vi "GetPatternMatchResultValue.vi"(8 "error in (no error)":errorcluster, 9 "PatternMatchResult":T1 {"results"."ROI Descriptor out"."Contours"."Type" items=["No Selection", "Point", "Line", "Rectangle", "Oval", "Polygon", "Freehand Region", "Annulus", "Unused2", "Unused3", "Broken Line", "Freehand Line", "Rotated Rectangle"]; "results"."Point"."Y" format="%.2f"; "results"."Point"."X" format="%.2f"; "results"."Rectangle"."Rotation" format="%.2f"; "results"."Rectangle"."Left" scale=0.0..1024.0; "results"."Rectangle"."Right" scale=0.0..1024.0}, 11 "PatternMatchParameter":T5={"Algorithm"=2, "Match Parameters"={"Number of Matches Requested"=1, "Minimum Match Score"=750.0, "Angle Ranges"=[]}, "ROI Descriptor"={"Global Rectangle"=[], "Contours"=[]}, "Advanced Options"=[{"Item"=1, "Value"=1.0}, {"Item"=103, "Value"=1.0}], "Template path"="", "XOffset"=0, "YOffset"=0} {"ROI Descriptor"."Contours"."Type" items=["No Selection", "Point", "Line", "Rectangle", "Oval", "Polygon", "Freehand Region", "Annulus", "Unused2", "Unused3", "Broken Line", "Freehand Line", "Rotated Rectangle"]; "Advanced Options"."Item" items=["LD Sampling - Minimum Constrast"=0, "LD Sampling - Enable Subpixel Accuracy"=1, "LD Sampling - Search Strategy"=2, "LD Sampling - Subpixel Iterations"=3, "LD Sampling - Subpixel Tolerance"=4, "LD Sampling - Initial Match List Length"=5, "LD Sampling - Match List Reduction Factor"=6, "LD Sampling - Initial Step Size"=7, "LD Sampling - Intermediate Angular Accuracy"=8, "-"=9, "Pyramid - Max Pyramid Level"=100, "Pyramid - Minimum Contrast"=102, "Pyramid - Enable Subpixel Accuracy"=103, "Pyramid - Subpixel Iterations"=104, "Pyramid - Subpixel Tolerance"=105, "Pyramid - Initial Match List Length"=106, "Pyramid - Match List Reduction Factor"=107, "Pyramid - Intermediate Angular Accuracy"=108, "Pyramid - Process Border Matches"=109, "Pyramid - Min Match Separation Distance"=111, "Pyramid - Min Match Separation Angle"=112, "Pyramid - Max Match Overlap"=113, "Pyramid - Max Cache in MB"=114, "Pyramid - Clear Cache"=115]; "Match Parameters"."Angle Ranges"."End Angle" min=-360 max=360; "Match Parameters"."Angle Ranges"."Start Angle" min=-360 max=360; "Match Parameters"."Minimum Match Score" min=0 max=1000; "Match Parameters"."Number of Matches Requested" min=1 max=9999; "Algorithm" items=["All", "Low Discrepancy Sampling", "Grayscale Value Pyramid", "Gradients Pyramid"]}) -> (0 "error out":errorcluster, 3 "ResultValues":string[](array[string]))   [LabVIEW 2019]
uses:
  Controls/Parttern Match/Analysis_PatternMatch_Parameter.ctl
  Controls/Parttern Match/Analysis_PatternMatch_ResultWithnumber.ctl
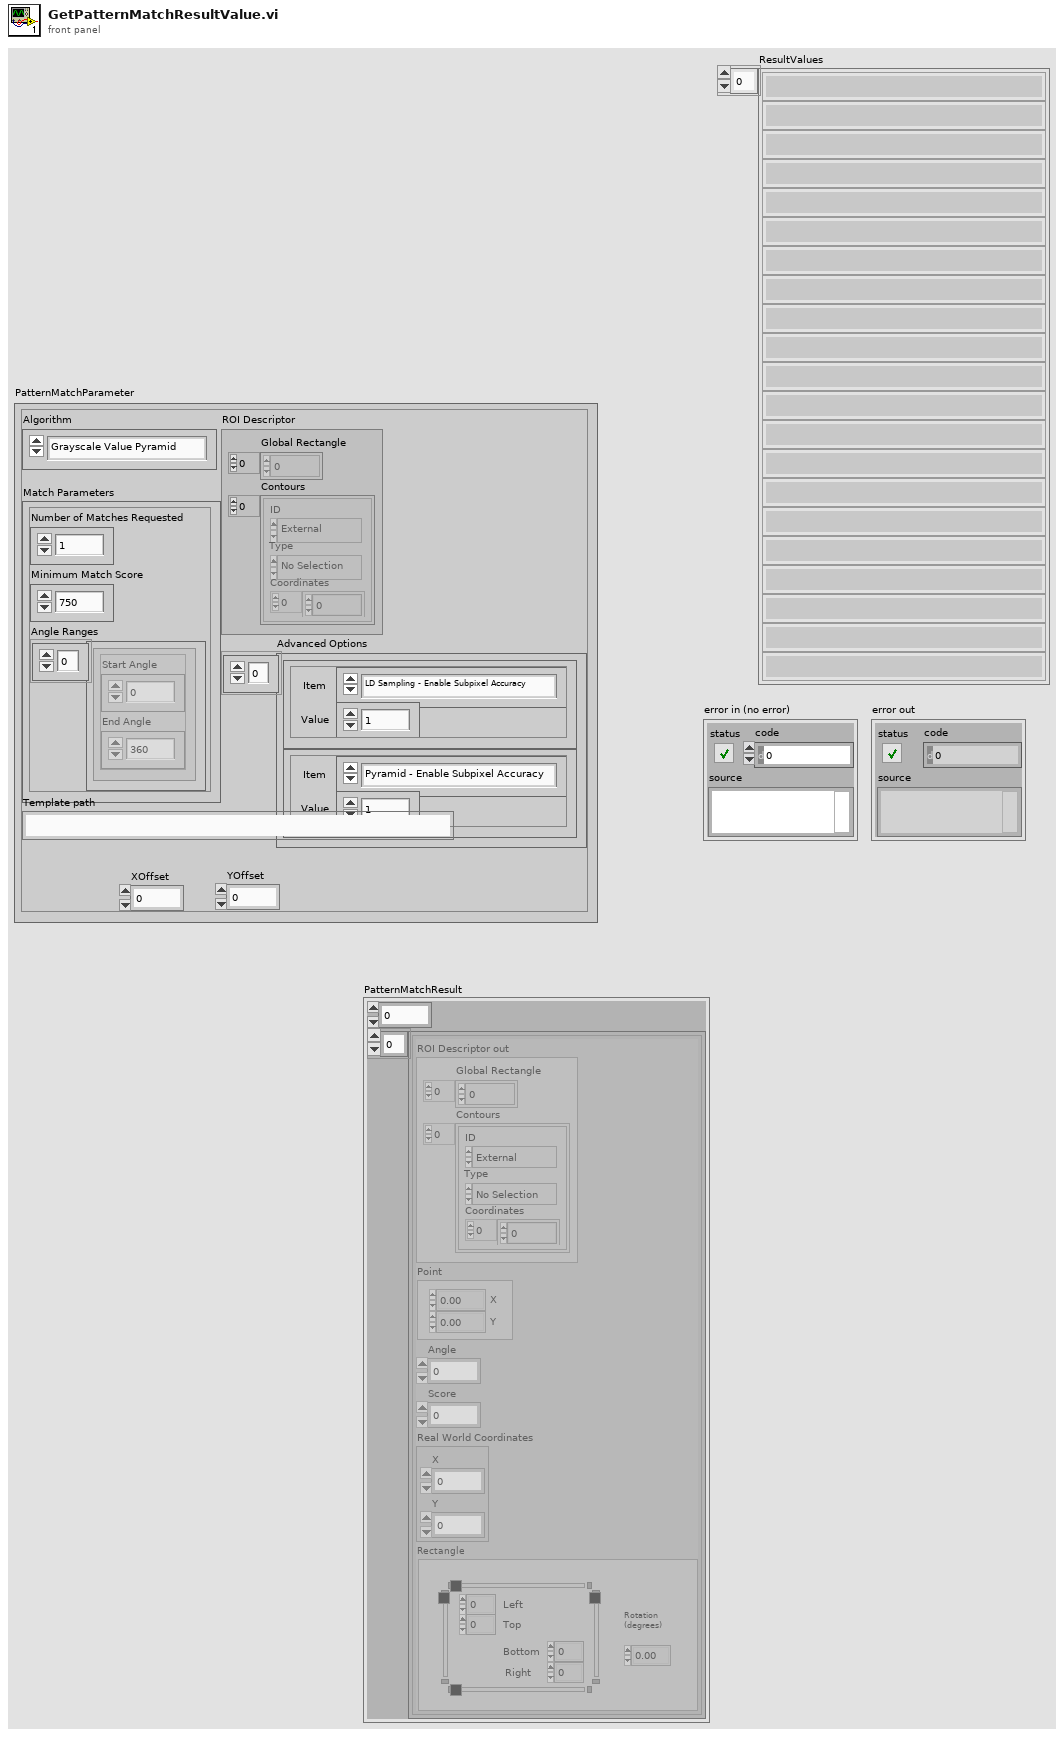
[diagram p1: front panel]
types:
  T1 = typedef "Analysis_PatternMatch_ResultWithnumber.ctl" = cluster{"numbers":i32, "results":cluster{"ROI Descriptor out":T2, "Point":T3, "Angle":sgl, "Score":sgl, "Real World Coordinates":cluster{"X":sgl, "Y":sgl}, "Rectangle":T4}[]}
  T2 = typedef "ROI Descriptor" = cluster{"Global Rectangle":i32[], "Contours":cluster{"ID":enum32{"External", "Internal"}, "Type":u32, "Coordinates":i32[]}[]}
  T3 = typedef "IMAQ Point" = cluster{"X":sgl, "Y":sgl}
  T4 = typedef "IMAQ Rectangle" = cluster{"Left":i32, "Top":i32, "Right":i32, "Bottom":i32, "Rotation":dbl}
  T5 = typedef "Analysis_PatternMatch_Parameter.ctl" = cluster{"Algorithm":i32, "Match Parameters":cluster{"Number of Matches Requested":i32, "Minimum Match Score":sgl, "Angle Ranges":cluster{"Start Angle":sgl, "End Angle":sgl}[]}, "ROI Descriptor":T2, "Advanced Options":cluster{"Item":u16, "Value":dbl}[], "Template path":string, "XOffset":i32, "YOffset":i32}
  T6 = cluster{"ROI Descriptor out":T2, "Point":T3, "Angle":sgl, "Score":sgl, "Real World Coordinates":cluster{"X":sgl, "Y":sgl}, "Rectangle":T4}[]
  T7 = cluster{"ROI Descriptor out":T2, "Point":T3, "Angle":sgl, "Score":sgl, "Real World Coordinates":cluster{"X":sgl, "Y":sgl}, "Rectangle":T4}
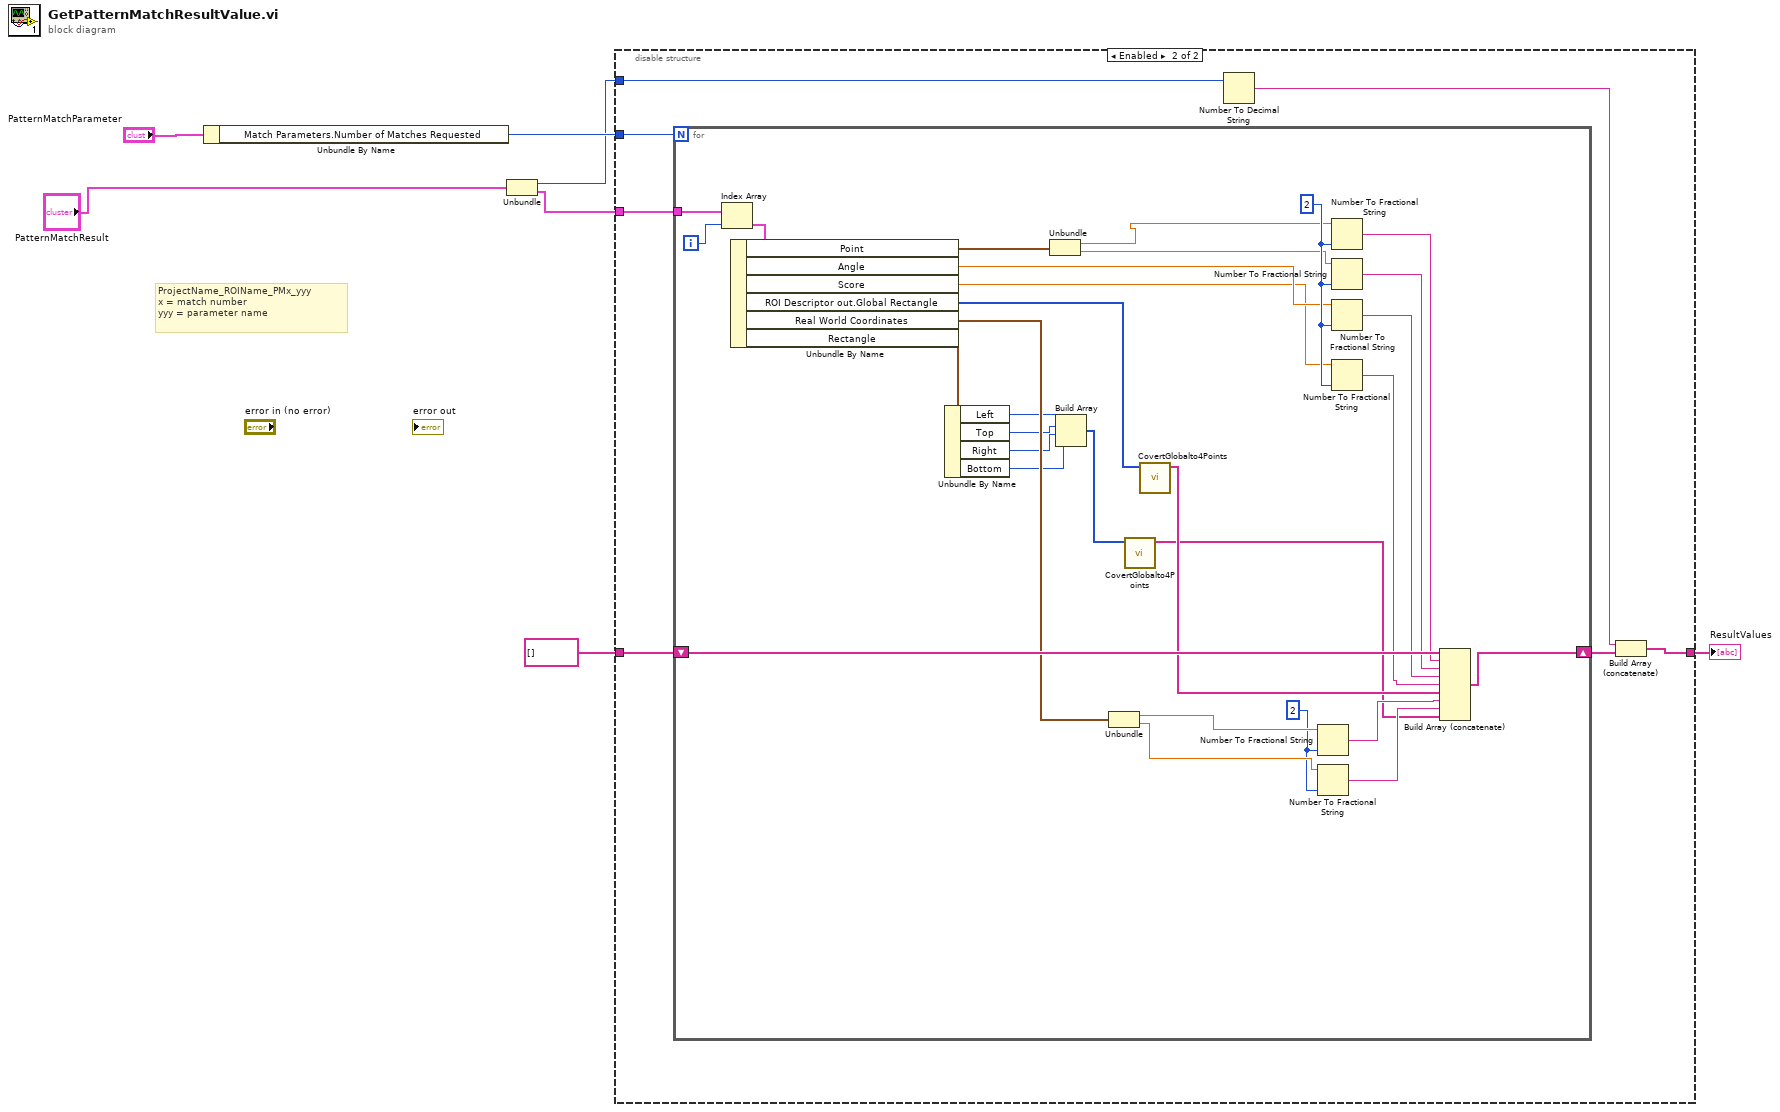
[diagram p0: block diagram]
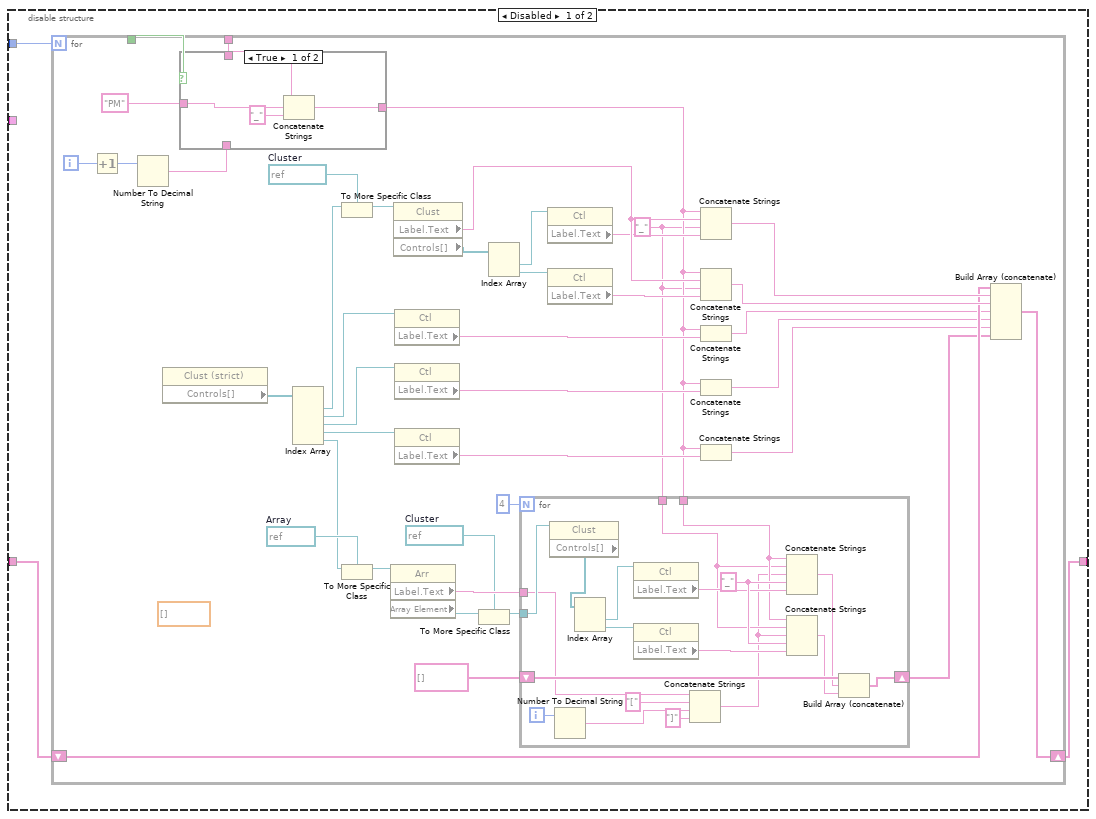
[diagram p2: hidden frame]
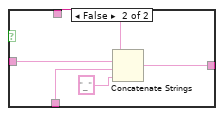
[diagram p3: hidden frame]
diagram:
  # "ProjectName_ROIName_PMx_yyy\nx = match number\nyyy = parameter name"
  n1 = Unbundle By Name("PatternMatchParameter") -> ("Match Parameters.Number of Matches Requested"=w6:i32)
  n2 = Unbundle("PatternMatchResult") -> ("numbers"=w1:i32, "results"=w2:T6)
  n3 = disable-structure shown="Enabled" {
    disable-tunnel: w6 -> [w11 w88]
    disable-tunnel: string[] [] -> [w10 w87]
    disable-tunnel: [w9 w84] -> w4
    disable-tunnel: w2 -> [_ w85]
    disable-tunnel: w1 -> [_ w83]
    frame Disabled {
      n4 = for {
        N: w11 -> [_]
        tunnel: _ -> [w33]
        shift-right: [w35] -> w9
        shift-left: w10 -> [w36]
        tunnel: [w34] -> w8
        i -> [w39]
        w18 = refnum<vi> refnum  # Cluster
        (unwired) dbl[] []
        w23 = refnum<vi> refnum  # Array
        w14 = "_" ("string")
        w49 = refnum<vi> refnum  # Cluster
        n5 = Increment(x=w39) -> (x+1=w38:i32)
        n6 = Number To Decimal String(number=w38) -> (decimal integer string=w32:string)  [unwired: 1 in]
        n7 = property class="Clust (strict)"() -> (reference=w53:refnum<vi>, "Controls[]"=w52:refnum<vi>[])  [unwired: 1 in, 2 out]
        n8 = case shown="True" w34 {
          tunnel: w33 -> [w76 w81]
          tunnel: w32 -> [_ w78]
          tunnel: [w75 w80] -> w15
          tunnel: "PM" ("string") -> [w74 w77]
          frame True {
            n9 = Concatenate Strings(w76, w74, "_" ("string")) -> (w75:string)
          }
          frame False {
            n10 = Concatenate Strings(w81, w77, w78, "_" ("string")) -> (w80:string)
          }
        }
        n11 = Index Array(array=w52) -> (element #1=w51:refnum<vi>, element #2=w30:refnum<vi>, element #3=w29:refnum<vi>, element #4=w42:refnum<vi>, element #5=w22:refnum<vi>)  [unwired: 5 in]
        n12 = To More Specific Class(target class=w49, reference=w51) -> (specific class reference=w50:refnum<vi>)  [unwired: 1 in, 1 out]
        n13 = To More Specific Class(target class=w23, reference=w22) -> (specific class reference=w21:refnum<vi>)  [unwired: 1 in, 1 out]
        n14 = property class="Arr"(reference=w21) -> ("Label.Text"=w20:string, "Array Element"=w17:refnum<vi>)  [unwired: 1 in, 2 out]
        n15 = property class="Clust"(reference=w50) -> ("Label.Text"=w45:string, "Controls[]"=w48:refnum<vi>[])  [unwired: 1 in, 2 out]
        n16 = property class="Ctl"(reference=w30) -> ("Label.Text"=w28:string)  [unwired: 1 in, 2 out]
        n17 = property class="Ctl"(reference=w29) -> ("Label.Text"=w27:string)  [unwired: 1 in, 2 out]
        n18 = property class="Ctl"(reference=w42) -> ("Label.Text"=w37:string)  [unwired: 1 in, 2 out]
        n19 = To More Specific Class(target class=w18, reference=w17) -> (specific class reference=w16:refnum<vi>)  [unwired: 1 in, 1 out]
        n20 = Index Array(array=w48) -> (element #1=w47:refnum<vi>, element #2=w46:refnum<vi>)  [unwired: 2 in]
        n21 = for {
          N: 4 -> [_]
          tunnel: w20 -> [w58]
          tunnel: w16 -> [w72]
          tunnel: w15 -> [w65]
          tunnel: w14 -> [w64]
          shift-right: [w60] -> w12
          shift-left: string[] [] -> [w63]
          i -> [w59]
          w71 = "_" ("string")
          n22 = property class="Clust"(reference=w72) -> ("Controls[]"=w66:refnum<vi>[])  [unwired: 1 in, 2 out]
          n23 = Number To Decimal String(number=w59) -> (decimal integer string=w56:string)  [unwired: 1 in]
          n24 = Index Array(array=w66) -> (element #1=w67:refnum<vi>, element #2=w68:refnum<vi>)  [unwired: 2 in]
          n25 = property class="Ctl"(reference=w67) -> ("Label.Text"=w69:string)  [unwired: 1 in, 2 out]
          n26 = property class="Ctl"(reference=w68) -> ("Label.Text"=w70:string)  [unwired: 1 in, 2 out]
          n27 = Concatenate Strings(w58, "[" ("string"), w56, "]" ("string")) -> (w54:string)
          n28 = Concatenate Strings(w65, w64, w54, w71, w69) -> (w62:string)
          n29 = Concatenate Strings(w65, w64, w54, w71, w70) -> (w61:string)
          n30 = Build Array (concatenate)(w63, w62, w61) -> (w60:string[])
        }
        n31 = property class="Ctl"(reference=w47) -> ("Label.Text"=w44:string)  [unwired: 1 in, 2 out]
        n32 = property class="Ctl"(reference=w46) -> ("Label.Text"=w43:string)  [unwired: 1 in, 2 out]
        n33 = Concatenate Strings(w15, w45, w14, w44) -> (w41:string)
        n34 = Concatenate Strings(w15, w45, w14, w43) -> (w40:string)
        n35 = Concatenate Strings(w15, w28) -> (w24:string)
        n36 = Concatenate Strings(w15, w27) -> (w25:string)
        n37 = Concatenate Strings(w15, w37) -> (w26:string)
        n38 = Build Array (concatenate)(w36, w41, w40, w24, w25, w26, w12) -> (w35:string[])
      }
    }
    frame Enabled {
      n39 = for {
        N: w88 -> [_]
        shift-right: [w107] -> w86
        shift-left: w87 -> [w111]
        tunnel: w85 -> [w118]
        i -> [w117]
        w98 = i16 2 ("precision (6)")
        w114 = i16 2 ("precision (6)")
        n40 = Index Array(array=w118, index=w117) -> (element=w116:T7)
        n41 = Unbundle By Name(w116) -> ("Point"=w106:T3, "Angle"=w113:sgl, "Score"=w112:sgl, "ROI Descriptor out.Global Rectangle"=w115:i32[], "Real World Coordinates"=w101:cluster{"X":sgl, "Y":sgl}, "Rectangle"=w95:T4)
        n42 = Unbundle By Name(w95) -> ("Left"=w94:i32, "Top"=w93:i32, "Right"=w92:i32, "Bottom"=w91:i32)
        n43 = Unbundle(w106) -> ("X"=w104:sgl, "Y"=w105:sgl)
        n44 = Build Array(w94, w93, w92, w91) -> (w90:i32[])
        n45 = Unbundle(w101) -> ("X"=w100:sgl, "Y"=w99:sgl)
        n46 = call "CovertGlobalto4Points.vi"("Global Rectangle"=w90) -> ("Array"=w89:string[])  [unwired: 10 in]
        n47 = call "CovertGlobalto4Points.vi"("Global Rectangle"=w115) -> ("Array"=w102:string[])  [unwired: 10 in]
        n48 = Number To Fractional String(number=w100, precision (6)=w98) -> (F-format string=w97:string)  [unwired: 2 in]
        n49 = Number To Fractional String(number=w99, precision (6)=w98) -> (F-format string=w96:string)  [unwired: 2 in]
        n50 = Number To Fractional String(number=w104, precision (6)=w114) -> (F-format string=w110:string)  [unwired: 2 in]
        n51 = Number To Fractional String(number=w105, precision (6)=w114) -> (F-format string=w109:string)  [unwired: 2 in]
        n52 = Number To Fractional String(number=w113, precision (6)=w114) -> (F-format string=w108:string)  [unwired: 2 in]
        n53 = Number To Fractional String(number=w112, precision (6)=w114) -> (F-format string=w103:string)  [unwired: 2 in]
        n54 = Build Array (concatenate)(w111, w110, w109, w108, w103, w102, w97, w96, w89) -> (w107:string[])
      }
      n55 = Number To Decimal String(number=w83) -> (decimal integer string=w82:string)  [unwired: 1 in]
      n56 = Build Array (concatenate)(w82, w86) -> (w84:string[])
    }
  }
  "ResultValues" <- w4
